vi "Digitial Integrator Read Gain.vi"(8 "error in (no error)":errorcluster, 11 "VISA resource name":refnum<visa-resource-name>) -> (0 "error out":errorcluster, 2 "Gain":i16(slide)=1 min=0 max=9 step=1 scale=0.0..9.0, 3 "VISA resource name dup":refnum<visa-resource-name>)   [LabVIEW 2025]
doc: "Author: Scott Hannahs <sth@magnet.fsu.edu>\n\nThis software is licensed for use under the “MIT License\"\nCopyright (c) 2025 Scott Hannahs, sth@sth@magnet.sthnet.net\n\nPermission is hereby granted, free of charge, to any person obtaining a copy of this software and associated documentation files (the \"Software\"), to deal in the Software without restriction, including without limitation the rights to use, copy, modify, merge, publish, distribute, sublicense, and/or sell copies of the Software, and to permit persons to whom the Software is furnished to do so, subject to the following conditions: The above copyright notice and this permission notice shall be included in all copies or substantial portions of the Software.\n\nTHE SOFTWARE IS PROVIDED \"AS IS\", WITHOUT WARRANTY OF ANY KIND, EXPRESS OR IMPLIED, INCLUDING BUT NOT LIMITED TO THE WARRANTIES OF MERCHANTABILITY, FITNESS FOR A PARTICULAR PURPOSE AND NONINFRINGEMENT. IN NO EVENT SHALL THE AUTHORS OR COPYRIGHT HOLDERS BE LIABLE FOR ANY CLAIM, DAMAGES OR OTHER LIABILITY, WHETHER IN AN ACTION OF CONTRACT, TORT OR OTHERWISE, ARISING FROM, OUT OF OR IN CONNECTION WITH THE SOFTWARE OR THE USE OR OTHER DEALINGS IN THE SOFTWARE."
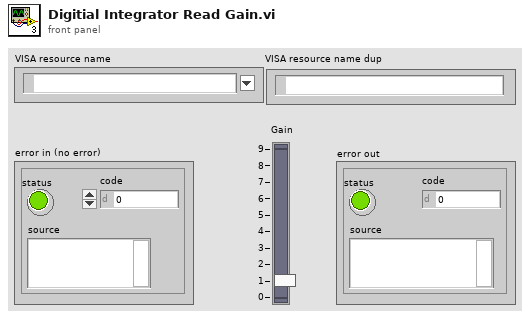
[diagram p1: front panel]
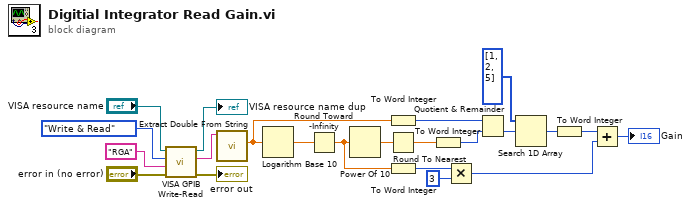
[diagram p0: block diagram]
diagram:
  n1 = call "VISA GPIB Write-Read.vi"("error in (no error)"="error in (no error)", "Command"="RGA" ("format string"), "Action"=enum16{"Write", "Read", "Write & Read"}."Write & Read", "VISA resource name"="VISA resource name") -> ("error out"=→"error out":errorcluster, "String Returned"=w16:string, "dup VISA Session"=→"VISA resource name dup":refnum<visa-resource-name>)  [unwired: 4 in, 1 out]
  n2 = call "Extract Double From String.vi"("string"=w16) -> ("floating pt. number"=w12:dbl)  [unwired: 3 in, 3 out]
  n3 = Logarithm Base 10(1:w12) -> (0:w15:dbl)
  n4 = Round Toward -Infinity(1:w15) -> (0:w14:dbl)
  n5 = Power Of 10(x=w14) -> (10^x=w13:dbl)
  n6 = To Word Integer(number=w12) -> (16bit integer=w11:i16)
  n7 = Round To Nearest(number=w13) -> (nearest integer value=w10:dbl)
  n8 = To Word Integer(number=w14) -> (16bit integer=w6:i16)
  n9 = To Word Integer(number=w10) -> (16bit integer=w9:i16)
  n10 = Multiply(x=w6, y=i16 3) -> (x*y=w3:i16)
  n11 = Quotient & Remainder(x=w11, y=w9) -> (floor(x/y)=w7:i16)  [unwired: 1 out]
  n12 = Search 1D Array(1D array=i16[] [1, 2, 5] ("array"), element=w7) -> (index of element=w4:i32)  [unwired: 1 in]
  n13 = To Word Integer(number=w4) -> (16bit integer=w1:i16)
  n14 = Add(x=w1, y=w3) -> (x+y=→"Gain":i16)
